vi "dfd_Maxflat Find Order.vi"(7 "symmetric FIR ? (T)":bool, 8 "error in (no error)":errorcluster, 9 "normalized fc":dbl=0.2, 10 "denominator order":i32=2, 11 "numerator order":i32=2) -> (0 "error out":errorcluster, 1 "N":i32=2, 2 "M":i32=1, 3 "L":i32=3)   [LabVIEW 2017, in "NI_DigFilter_Design.lvlib"]
doc: "Gets the number of zeros at z = -1 \"<B>L</B>\", remaining zeros \"<B>M</B>\", and poles of the filter \"<B>N</B>\"."
uses:
  <vilib>/addons/Digital Filter Design/NI_DigFilter_Design.lvlib
  <vilib>/addons/Digital Filter Design/_Misc.llb/dfd_Error Handlers (Single).vi
  <vilib>/addons/Digital Filter Design/NI_DigFilterLicensed.lvlib
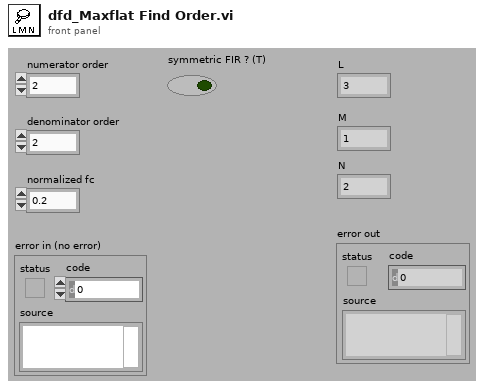
[diagram p1: front panel]
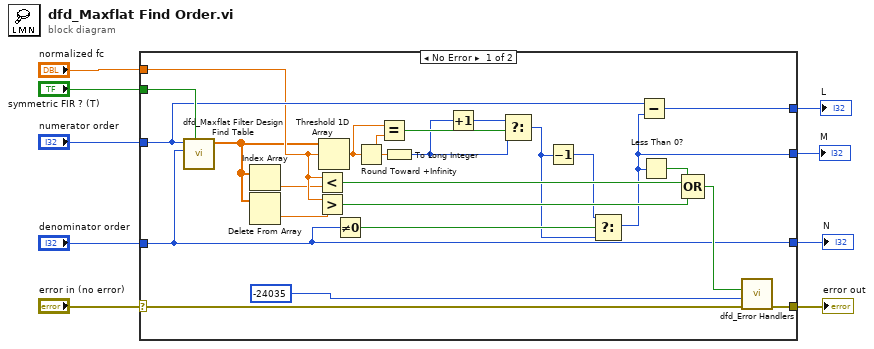
[diagram p0: block diagram]
diagram:
  n1 = case shown="No Error" "error in (no error)" {
    selector: "error in (no error)" -> [w31 w34]
    tunnel: "symmetric FIR ? (T)" -> [w33 _]
    tunnel: [w32 w34] -> w8
    tunnel: "numerator order" -> [w29 _]
    tunnel: "denominator order" -> [w19 _]
    tunnel: [w17 _] -> w2
    tunnel: [w28 _] -> w1
    tunnel: [w19 _] -> w5
    tunnel: "normalized fc" -> [w27 _]
    frame No Error {
      n2 = call <vilib>:"dfd_Maxflat Filter Design Find Table.vi"("symmetric FIR ? (T)"=w33, "denominator order"=w19, "numerator order"=w29) -> ("table"=w25:dbl[])  [unwired: 8 out]
      n3 = Index Array(array=w25) -> (element=w26:dbl)  [unwired: 1 in]
      n4 = Delete From Array(array=w25) -> (deleted portion=w24:dbl)  [unwired: 2 in, 1 out]
      n5 = Less?(x=w27, y=w26) -> (x < y?=w23:bool)
      n6 = Greater?(x=w27, y=w24) -> (0:w22:bool)
      n7 = Threshold 1D Array(2:w27, 3:w25) -> (0:w15:dbl)  [unwired: 1 out]
      n8 = Not Equal To 0?(x=w19) -> (x != 0?=w18:bool)
      n9 = Round Toward +Infinity(x=w15) -> (ceil(x): smallest int >= x=w16:dbl)
      n10 = Equal?(x=w15, y=w16) -> (x = y?=w13:bool)
      n11 = To Long Integer(number=w16) -> (32bit integer=w11:i32)
      n12 = Increment(x=w11) -> (x+1=w12:i32)
      n13 = Select(t=w12, s=w13, f=w11) -> (s? t:f=w10:i32)
      n14 = Decrement(x=w10) -> (x-1=w14:i32)
      n15 = Select(t=w14, s=w18, f=w10) -> (s? t:f=w17:i32)
      n16 = Subtract(x=w29, y=w17) -> (x-y=w28:i32)
      n17 = Less Than 0?(x=w17) -> (x < 0?=w20:bool)
      n18 = Compound Arithmetic op=OR(w20, w23, w22) -> (w21:bool)
      n19 = call-poly <vilib>:"dfd_Error Handlers.vi"("error in (no error)"=w31, "error code"=-24035 ("ERR_FILTER_DESIGN_FAIL"), "condition failed?"=w21) -> ("error out"=w32:errorcluster)  [unwired: 8 out]
    }
    frame Error {
    }
  }
  "L" <- w1
  "M" <- w2
  "N" <- w5
  "error out" <- w8
